vi "DAQ_Init.vi"(8 "error in":errorcluster caption="entrée d'erreur") -> (0 "error out":errorcluster caption="sortie d'erreur")   [LabVIEW 2026]
uses:
  FGV/FGV_DAQ_CO_Task.vi
  Controls/TypeDef_FGV.ctl
  <vilib>/DAQmx/create/channels.llb/DAQmx Create Channel (CO-Pulse Generation-Time).vi
  <vilib>/DAQmx/configure/timing.llb/DAQmx Timing (Implicit).vi
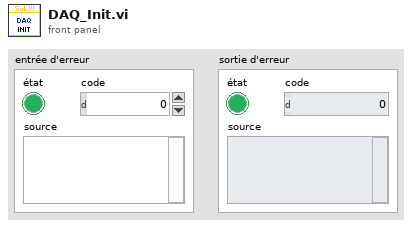
[diagram p1: front panel]
types:
  T1 = typedef "TypeDef_FGV.ctl" = enum16{"Initialize", "Write", "Read"}
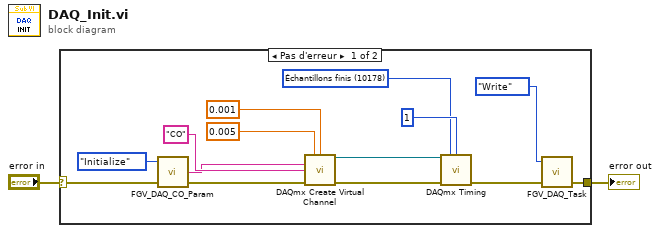
[diagram p0: block diagram]
diagram:
  n1 = case shown="Pas d'erreur" "error in" {
    selector: "error in" -> [w13 w17]
    tunnel: [w15 w17] -> w1
    frame No Error {
      w3 = 10178 items=["Échantillons finis"=10178, "Échantillons continus"=10123, "Point par point avec cadencement matériel"=12522] ("sample mode")
      n2 = call "FGV_DAQ_CO_Param.vi"("error in"=w13, "Action"=TypeDef_FGV."Initialize") -> ("error out"=w12:errorcluster, "CO line"=w10:tag)  [unwired: 2 in]
      n3 = call-poly <vilib>:"DAQmx Create Virtual Channel.vi"("high time"=0.005, "low time"=0.001, "counter"=w10, "name to assign"="CO", "error in"=w12) -> ("task out"=w7:refnum<k21>, "error out"=w6:errorcluster)  [unwired: 9 in]
      n4 = call-poly <vilib>:"DAQmx Timing.vi"("task/channels in"=w7, "sample mode"=w3, "samples per channel"=1, "error in"=w6) -> ("error out"=w5:errorcluster)  [unwired: 10 in, 1 out]
      n5 = call "FGV_DAQ_Task.vi"("error in"=w5, "Action"=TypeDef_FGV."Write") -> ("error out"=w15:errorcluster)  [unwired: 2 in, 1 out]
    }
    frame Error {
    }
  }
  "error out" <- w1
